vi "SQLFetch.vi"(4 "error in (no error)":errorcluster, 7 "InputHandle":i32) -> (0 "error out":errorcluster, 2 "Data Present?":bool, 3 "OutputHandle":i32)   [LabVIEW 2011]
doc: "Charge la prochaine ligne de résultat"
uses:
  Odbc32.dll
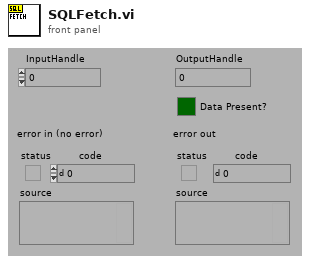
[diagram p1: front panel]
types:
  T1 = enum16{"NOPE", "SQL_HANDLE_ENV", "SQL_HANDLE_DBC", "SQL_HANDLE_STMT", "SQL_HANDLE_DESC"}
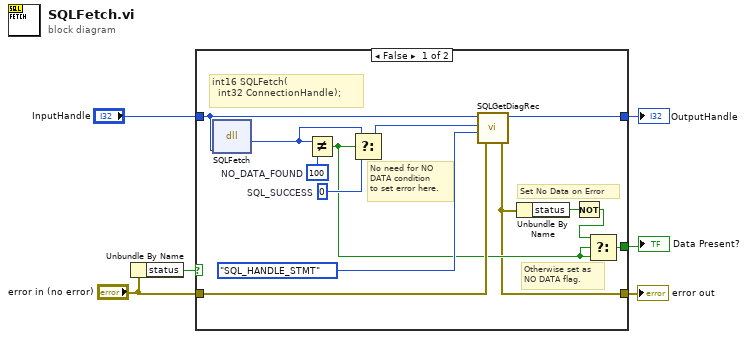
[diagram p0: block diagram]
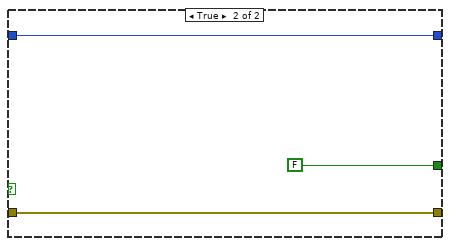
[diagram p2: hidden frame]
diagram:
  n1 = Unbundle By Name("error in (no error)") -> ("status"=w4:bool)
  n2 = case shown="False" w4 {
    tunnel: "InputHandle" -> [w19 w21]
    tunnel: [w17 w21] -> w5
    tunnel: "error in (no error)" -> [w18 w22]
    tunnel: [w9 w22] -> w2
    tunnel: [w11 FALSE] -> w1
    frame False {
      w12 = i16 0  # SQL_SUCCESS
      w15 = i16 100  # NO_DATA_FOUND
      # "Otherwise set as\nNO DATA flag."
      # "Set No Data on Error"
      # "No need for NO \nDATA condition\nto set error here."
      # "int16 SQLFetch(\n  int32 ConnectionHandle);"
      n3 = dll-call lib="Odbc32.dll" fn="SQLFetch"("ConnectionHandle"=w19) -> (w13:i16)  [unwired: 4 in, 2 out]
      n4 = Not Equal?(x=w13, y=w15) -> (x != y?=w10:bool)
      n5 = Select(t=w13, s=w10, f=w12) -> (s? t:f=w14:i16)
      n6 = call "SQLGetDiagRec.vi"("error in (no error)"=w18, "HandleType"=T1."SQL_HANDLE_STMT", "Status (SQL_SUCCESS=0)"=w14, "Input Handle"=w19) -> ("error out"=w9:errorcluster, "Output Handle"=w17:i32)  [unwired: 2 out]
      n7 = Unbundle By Name(w9) -> ("status"=w8:bool)
      n8 = Not(x=w8) -> (.not. x?=w7:bool)
      n9 = Select(t=w7, s=w10, f=w10) -> (s? t:f=w11:bool)
    }
    frame True {
    }
  }
  "OutputHandle" <- w5
  "error out" <- w2
  "Data Present?" <- w1
